vi "2ballzautogood.vi"() -> (3 "Outputs":T1)   [LabVIEW 2013]
uses:
  outputs.ctl
  drive/drive_outputs.ctl
  flinger/flinger_outputs.ctl
  <vilib>/Rock Robotics/WPI/Solenoid/WPI_SolenoidValue.ctl
  roller/roller_outputs.ctl
  catch/catch_outputs.ctl
  inputs.ctl
  drive/drive_inputs.ctl
  flinger/flinger_inputs.ctl
  roller/roller_inputs.ctl
  catch/catch_inputs.ctl
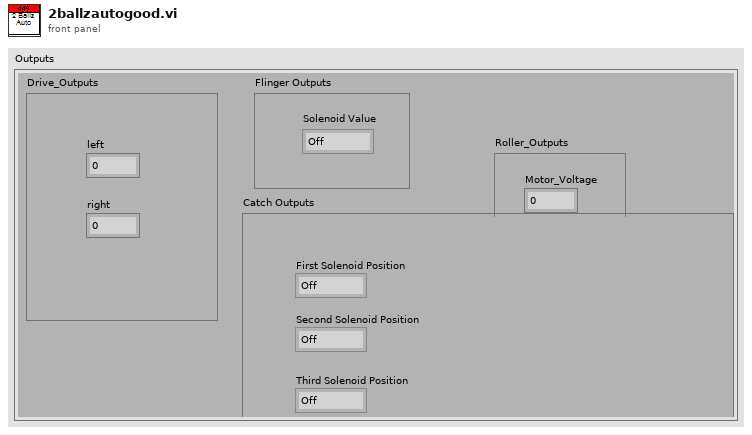
[diagram p1: front panel]
types:
  T1 = typedef "outputs.ctl" = cluster{"Drive_Outputs":T2, "Flinger Outputs":T3, "Roller_Outputs":T5, "Catch Outputs":T6}
  T2 = typedef "drive_outputs.ctl" = cluster{"left":dbl, "right":dbl}
  T3 = typedef "flinger_outputs.ctl" = cluster{"Solenoid Value":T4}
  T4 = typedef "WPI_SolenoidValue.ctl" = enum16{"Off", "On", "Forward", "Reverse"}
  T5 = typedef "roller_outputs.ctl" = cluster{"Sol_Position":T4, "Motor_Voltage":dbl}
  T6 = typedef "catch_outputs.ctl" = cluster{"First Solenoid Position":T4, "Second Solenoid Position":T4, "Third Solenoid Position":T4}
  T7 = enum16{"zero", "first", "second", "third", "fourth", "fifth", "sixth", "seventh", "eighth", "ninth"}
  T8 = typedef "WPI_EncoderDevRef.ctl" = cluster{"DevStatus":errorcluster, "EncoderIndex":T9, "CounterIndex":T10, "DistancePerCount":dbl, "Decoding Type":T11}
  T9 = typedef "FPGA_EncoderIdx.ctl" = enum8{"Enc 0", "Enc 1", "Enc 2", "Enc 3", "Invalid"}
  T10 = typedef "FPGA_CounterCtrSystemIndex.ctl" = enum8{"Ctr 0", "Ctr 1", "Ctr 2", "Ctr 3", "Ctr 4", "Ctr 5", "Ctr 6", "Ctr 7", "Invalid"}
  T11 = typedef "WPI_EncoderType.ctl" = enum16{"1x", "2x", "4x"}
  T12 = typedef "inputs.ctl" = cluster{"Drive_inputs":T13, "Flinger Inputs":T14, "Roller Inputs":T15, "Catch Inputs":T16}
  T13 = typedef "drive_inputs.ctl" = cluster{"j_x":dbl, "j_y":dbl, "Heading":dbl, "Left_Distance":dbl, " Right_Distance":dbl}
  T14 = typedef "flinger_inputs.ctl" = cluster{"Shoot":bool, "Power":dbl, "Safety":bool}
  T15 = typedef "roller_inputs.ctl" = cluster{"Arm_In":bool, "Full_Fore":bool, "Full_Back":bool, "Half_Fore":bool}
  T16 = typedef "catch_inputs.ctl" = cluster{"Default":bool, "Closed":bool, "Catch":bool, "Shoot":bool}
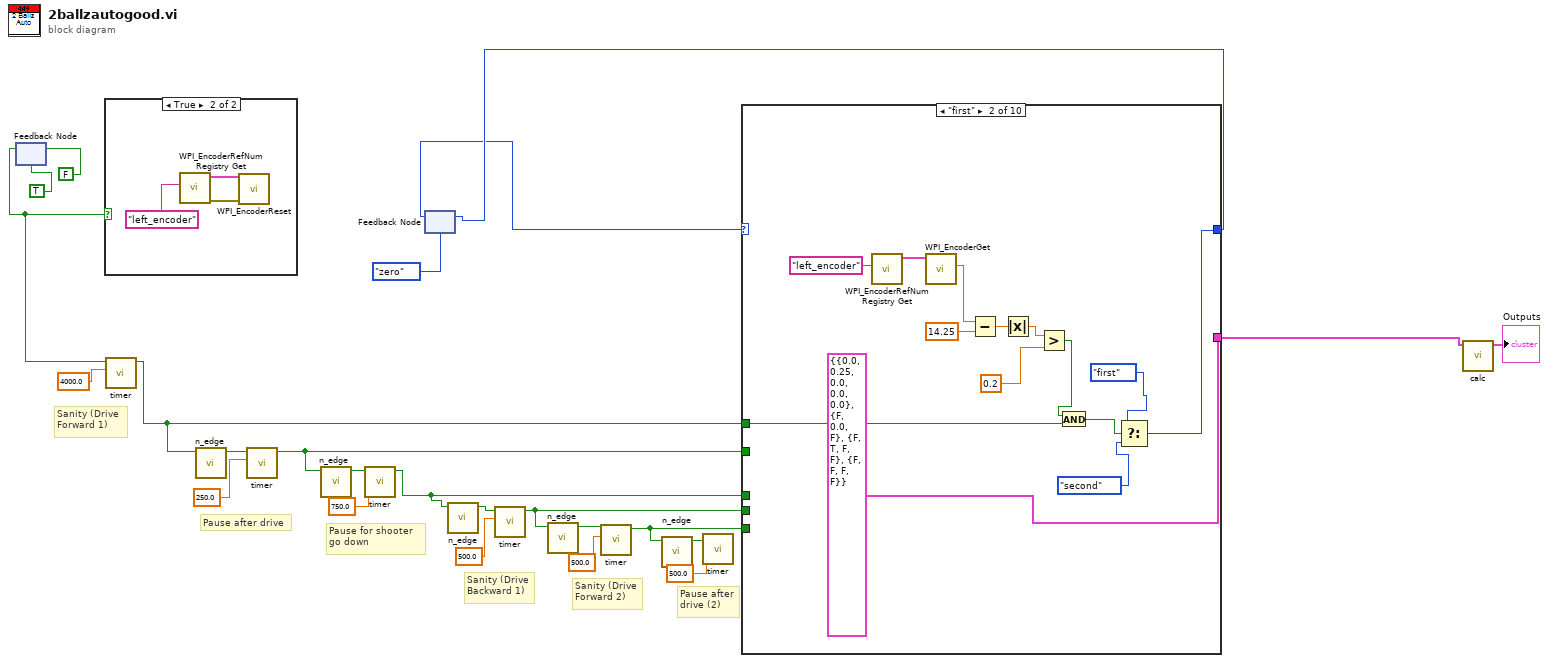
[diagram p0: block diagram]
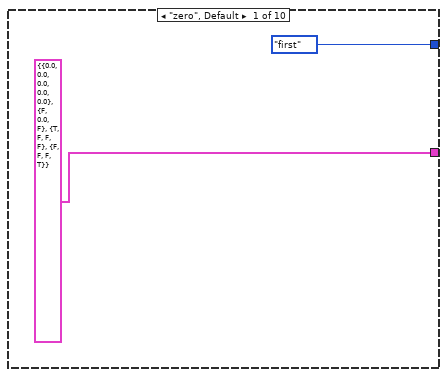
[diagram p2: hidden frame]
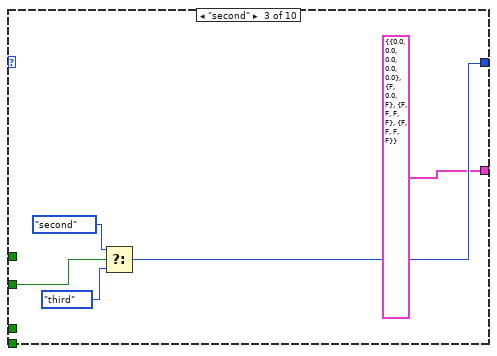
[diagram p3: hidden frame]
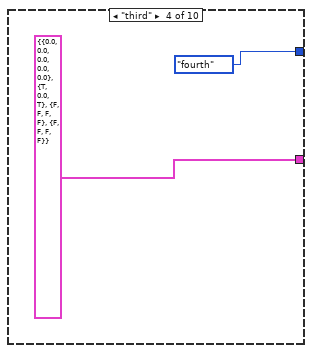
[diagram p4: hidden frame]
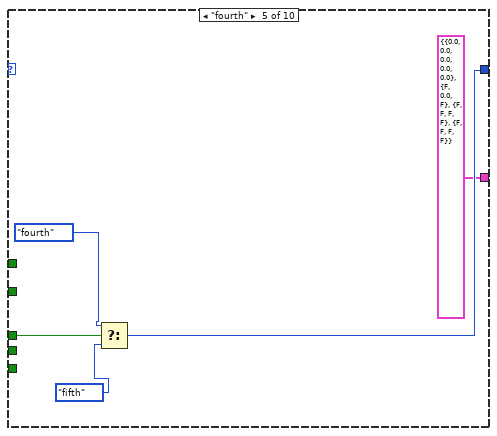
[diagram p5: hidden frame]
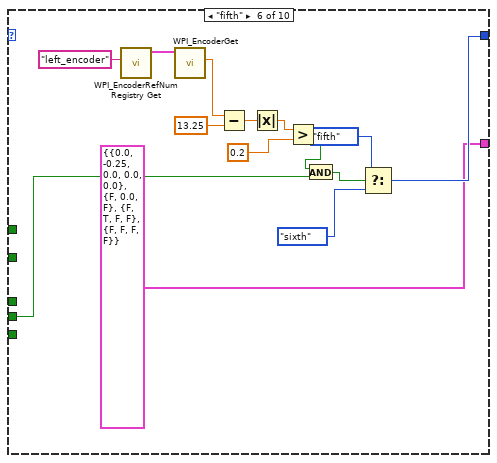
[diagram p6: hidden frame]
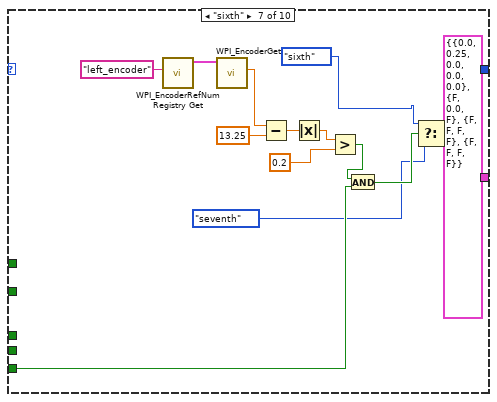
[diagram p7: hidden frame]
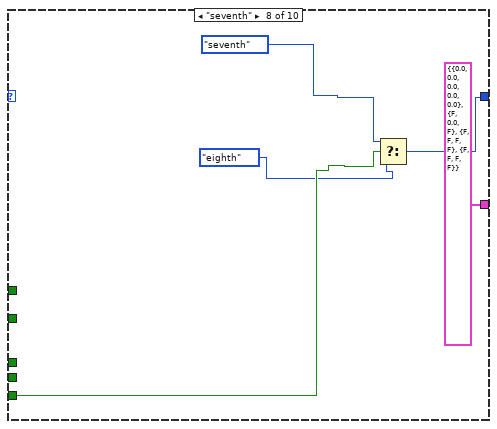
[diagram p8: hidden frame]
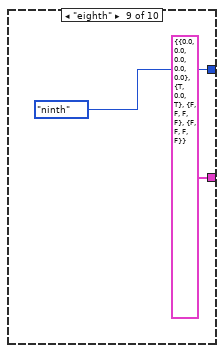
[diagram p9: hidden frame]
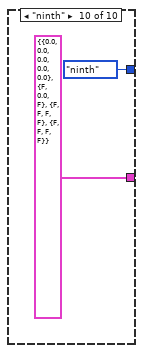
[diagram p10: hidden frame]
diagram:
  # "Pause after\ndrive (2)"
  # "Sanity (Drive\nForward 2)"
  # "Sanity (Drive\nBackward 1)"
  # "Pause for shooter \ngo down"
  # "Pause after drive"
  # "Sanity (Drive \nForward 1)"
  n1 = feedback-in #1(FALSE) -> ()
  n2 = feedback #1(TRUE) -> (w18:bool)
  n3 = case shown="True" w18 {
    frame False {
    }
    frame True {
      n4 = call <vilib>:"WPI_EncoderRefNum Registry Get.vi"("refnum name"="left_encoder") -> ("error out"=w26:errorcluster, "EncoderDevRef"=w27:T8)  [unwired: 9 in]
      n5 = call <vilib>:"WPI_EncoderReset.vi"("error in (no error)"=w26, "EncoderDevRef"=w27) -> ()  [unwired: 8 in, 2 out]
    }
  }
  n6 = call "timer.vi"("Time"=4000.0, "Set"=w18) -> ("Out"=w16:bool)  [unwired: 9 in]
  n7 = call "n_edge.vi"("In"=w16) -> ("Out"=w15:bool)  [unwired: 10 in]
  n8 = call "timer.vi"("Time"=250.0, "Set"=w15) -> ("Out"=w12:bool)  [unwired: 9 in]
  n9 = call "n_edge.vi"("In"=w12) -> ("Out"=w10:bool)  [unwired: 10 in]
  n10 = call "timer.vi"("Time"=750.0, "Set"=w10) -> ("Out"=w9:bool)  [unwired: 9 in]
  n11 = feedback #2(T7."zero") -> (w13:T7)
  n12 = call "n_edge.vi"("In"=w9) -> ("Out"=w8:bool)  [unwired: 10 in]
  n13 = call "timer.vi"("Time"=500.0, "Set"=w8) -> ("Out"=w6:bool)  [unwired: 9 in]
  n14 = call "n_edge.vi"("In"=w6) -> ("Out"=w5:bool)  [unwired: 10 in]
  n15 = call "timer.vi"("Time"=500.0, "Set"=w5) -> ("Out"=w3:bool)  [unwired: 9 in]
  n16 = call "n_edge.vi"("In"=w3) -> ("Out"=w2:bool)  [unwired: 10 in]
  n17 = call "timer.vi"("Time"=500.0, "Set"=w2) -> ()  [unwired: 9 in, 1 out]
  n18 = case shown="\"first\"" w13 {
    tunnel: [T7."first" w33 w47 T7."fourth" w54 w59 w74 w88 T7."ninth" ("f") T7."ninth" ("f")] -> w20
    tunnel: [T12 {"Drive_inputs"={"j_x"=0.0, "j_y"=0.0, "Heading"=0.0, "Left_Distance"=0.0, " Right_Distance"=0.0}, "Flinger Inputs"={"Shoot"=FALSE, "Power"=0.0, "Safety"=FALSE}, "Roller Inputs"={"Arm_In"=TRUE, "Full_Fore"=FALSE, "Full_Back"=FALSE, "Half_Fore"=FALSE}, "Catch Inputs"={"Default"=FALSE, "Closed"=FALSE, "Catch"=FALSE, "Shoot"=TRUE}} ("Inputs") T12 {"Drive_inputs"={"j_x"=0.0, "j_y"=0.25, "Heading"=0.0, "Left_Distance"=0.0, " Right_Distance"=0.0}, "Flinger Inputs"={"Shoot"=FALSE, "Power"=0.0, "Safety"=FALSE}, "Roller Inputs"={"Arm_In"=FALSE, "Full_Fore"=TRUE, "Full_Back"=FALSE, "Half_Fore"=FALSE}, "Catch Inputs"={"Default"=FALSE, "Closed"=FALSE, "Catch"=FALSE, "Shoot"=FALSE}} ("Inputs") T12 {"Drive_inputs"={"j_x"=0.0, "j_y"=0.0, "Heading"=0.0, "Left_Distance"=0.0, " Right_Distance"=0.0}, "Flinger Inputs"={"Shoot"=FALSE, "Power"=0.0, "Safety"=FALSE}, "Roller Inputs"={"Arm_In"=FALSE, "Full_Fore"=FALSE, "Full_Back"=FALSE, "Half_Fore"=FALSE}, "Catch Inputs"={"Default"=FALSE, "Closed"=FALSE, "Catch"=FALSE, "Shoot"=FALSE}} ("Inputs") T12 {"Drive_inputs"={"j_x"=0.0, "j_y"=0.0, "Heading"=0.0, "Left_Distance"=0.0, " Right_Distance"=0.0}, "Flinger Inputs"={"Shoot"=TRUE, "Power"=0.0, "Safety"=TRUE}, "Roller Inputs"={"Arm_In"=FALSE, "Full_Fore"=FALSE, "Full_Back"=FALSE, "Half_Fore"=FALSE}, "Catch Inputs"={"Default"=FALSE, "Closed"=FALSE, "Catch"=FALSE, "Shoot"=FALSE}} ("Inputs") T12 {"Drive_inputs"={"j_x"=0.0, "j_y"=0.0, "Heading"=0.0, "Left_Distance"=0.0, " Right_Distance"=0.0}, "Flinger Inputs"={"Shoot"=FALSE, "Power"=0.0, "Safety"=FALSE}, "Roller Inputs"={"Arm_In"=FALSE, "Full_Fore"=FALSE, "Full_Back"=FALSE, "Half_Fore"=FALSE}, "Catch Inputs"={"Default"=FALSE, "Closed"=FALSE, "Catch"=FALSE, "Shoot"=FALSE}} ("Inputs") T12 {"Drive_inputs"={"j_x"=0.0, "j_y"=-0.25, "Heading"=0.0, "Left_Distance"=0.0, " Right_Distance"=0.0}, "Flinger Inputs"={"Shoot"=FALSE, "Power"=0.0, "Safety"=FALSE}, "Roller Inputs"={"Arm_In"=FALSE, "Full_Fore"=TRUE, "Full_Back"=FALSE, "Half_Fore"=FALSE}, "Catch Inputs"={"Default"=FALSE, "Closed"=FALSE, "Catch"=FALSE, "Shoot"=FALSE}} ("Inputs") T12 {"Drive_inputs"={"j_x"=0.0, "j_y"=0.25, "Heading"=0.0, "Left_Distance"=0.0, " Right_Distance"=0.0}, "Flinger Inputs"={"Shoot"=FALSE, "Power"=0.0, "Safety"=FALSE}, "Roller Inputs"={"Arm_In"=FALSE, "Full_Fore"=FALSE, "Full_Back"=FALSE, "Half_Fore"=FALSE}, "Catch Inputs"={"Default"=FALSE, "Closed"=FALSE, "Catch"=FALSE, "Shoot"=FALSE}} ("Inputs") T12 {"Drive_inputs"={"j_x"=0.0, "j_y"=0.0, "Heading"=0.0, "Left_Distance"=0.0, " Right_Distance"=0.0}, "Flinger Inputs"={"Shoot"=FALSE, "Power"=0.0, "Safety"=FALSE}, "Roller Inputs"={"Arm_In"=FALSE, "Full_Fore"=FALSE, "Full_Back"=FALSE, "Half_Fore"=FALSE}, "Catch Inputs"={"Default"=FALSE, "Closed"=FALSE, "Catch"=FALSE, "Shoot"=FALSE}} ("Inputs") T12 {"Drive_inputs"={"j_x"=0.0, "j_y"=0.0, "Heading"=0.0, "Left_Distance"=0.0, " Right_Distance"=0.0}, "Flinger Inputs"={"Shoot"=TRUE, "Power"=0.0, "Safety"=TRUE}, "Roller Inputs"={"Arm_In"=FALSE, "Full_Fore"=FALSE, "Full_Back"=FALSE, "Half_Fore"=FALSE}, "Catch Inputs"={"Default"=FALSE, "Closed"=FALSE, "Catch"=FALSE, "Shoot"=FALSE}} ("Inputs") T12 {"Drive_inputs"={"j_x"=0.0, "j_y"=0.0, "Heading"=0.0, "Left_Distance"=0.0, " Right_Distance"=0.0}, "Flinger Inputs"={"Shoot"=FALSE, "Power"=0.0, "Safety"=FALSE}, "Roller Inputs"={"Arm_In"=FALSE, "Full_Fore"=FALSE, "Full_Back"=FALSE, "Half_Fore"=FALSE}, "Catch Inputs"={"Default"=FALSE, "Closed"=FALSE, "Catch"=FALSE, "Shoot"=FALSE}} ("Inputs")] -> w19
    tunnel: w16 -> [_ w35 _ _ _ _ _ _ _ _]
    tunnel: w12 -> [_ _ w48 _ _ _ _ _ _ _]
    tunnel: w9 -> [_ _ _ _ w55 _ _ _ _ _]
    tunnel: w6 -> [_ _ _ _ _ w61 _ _ _ _]
    tunnel: w3 -> [_ _ _ _ _ _ w75 w86 _ _]
    frame "zero", Default {
    }
    frame "first" {
      n19 = call <vilib>:"WPI_EncoderRefNum Registry Get.vi"("refnum name"="left_encoder") -> ("EncoderDevRef"=w42:T8)  [unwired: 9 in, 1 out]
      n20 = call <vilib>:"WPI_EncoderGet.vi"("EncoderDevRef"=w42) -> ("Distance"=w41:dbl)  [unwired: 5 in, 5 out]
      n21 = Subtract(x=w41, y=14.25) -> (x-y=w39:dbl)
      n22 = Absolute Value(x=w39) -> (abs(x)=w38:dbl)
      n23 = Greater?(x=w38, y=0.2) -> (0:w36:bool)
      n24 = And(x=w36, y=w35) -> (x .and. y?=w34:bool)
      n25 = Select(t=T7."first", s=w34, f=T7."second") -> (s? t:f=w33:T7)
    }
    frame "second" {
      n26 = Select(t=T7."second", s=w48, f=T7."third") -> (s? t:f=w47:T7)
    }
    frame "third" {
    }
    frame "fourth" {
      n27 = Select(t=T7."fourth", s=w55, f=T7."fifth") -> (s? t:f=w54:T7)
    }
    frame "fifth" {
      n28 = call <vilib>:"WPI_EncoderRefNum Registry Get.vi"("refnum name"="left_encoder") -> ("EncoderDevRef"=w68:T8)  [unwired: 9 in, 1 out]
      n29 = call <vilib>:"WPI_EncoderGet.vi"("EncoderDevRef"=w68) -> ("Distance"=w67:dbl)  [unwired: 5 in, 5 out]
      n30 = Subtract(x=w67, y=13.25) -> (x-y=w65:dbl)
      n31 = Absolute Value(x=w65) -> (abs(x)=w64:dbl)
      n32 = Greater?(x=w64, y=0.2) -> (0:w62:bool)
      n33 = And(x=w62, y=w61) -> (x .and. y?=w60:bool)
      n34 = Select(t=T7."fifth", s=w60, f=T7."sixth") -> (s? t:f=w59:T7)
    }
    frame "sixth" {
      n35 = call <vilib>:"WPI_EncoderRefNum Registry Get.vi"("refnum name"="left_encoder") -> ("EncoderDevRef"=w82:T8)  [unwired: 9 in, 1 out]
      n36 = call <vilib>:"WPI_EncoderGet.vi"("EncoderDevRef"=w82) -> ("Distance"=w81:dbl)  [unwired: 5 in, 5 out]
      n37 = Subtract(x=w81, y=13.25) -> (x-y=w79:dbl)
      n38 = Absolute Value(x=w79) -> (abs(x)=w78:dbl)
      n39 = Greater?(x=w78, y=0.2) -> (0:w76:bool)
      n40 = And(x=w76, y=w75) -> (x .and. y?=w72:bool)
      n41 = Select(t=T7."sixth", s=w72, f=T7."seventh") -> (s? t:f=w74:T7)
    }
    frame "seventh" {
      n42 = Select(t=T7."seventh", s=w86, f=T7."eighth") -> (s? t:f=w88:T7)
    }
    frame "eighth" {
    }
    frame "ninth" {
    }
  }
  n43 = feedback-in #2(w20) -> ()
  n44 = call "calc.vi"("Inputs"=w19) -> ("Outputs"=→"Outputs":T1)  [unwired: 10 in]
